vi "Stop Work.vi"(8 "error in (no error)":errorcluster, 9 "Reply":bool=TRUE, 10 "Reply to":refnum<class "Stop Response Msg.lvclass">, 11 "Measure Object in":refnum<class "Instrument Actor.lvclass">) -> (0 "error out":errorcluster, 3 "Measure Object out":refnum<class "Instrument Actor.lvclass">)   [LabVIEW 2018, in "Instrument Actor.lvclass"]
uses:
  Instrument Actor.lvclass
  Controllers/Process Controller Messages/Stop Response Msg/Stop Response Msg.lvclass
  Instrument Actor.lvclass/Instrument Actor.ctl
  Read Instrument driver.vi
  Write Instrument driver.vi
  NHMFL_Core/Libraries/Instruments/Instrument Driver/Instrument Driver.lvclass
  Worker/Worker.lvclass
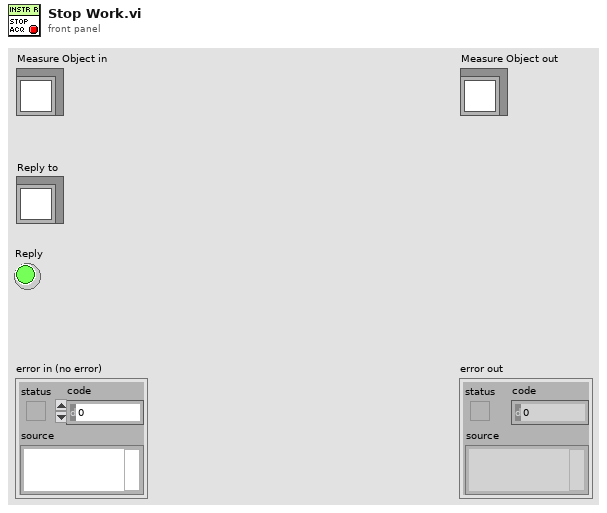
[diagram p1: front panel]
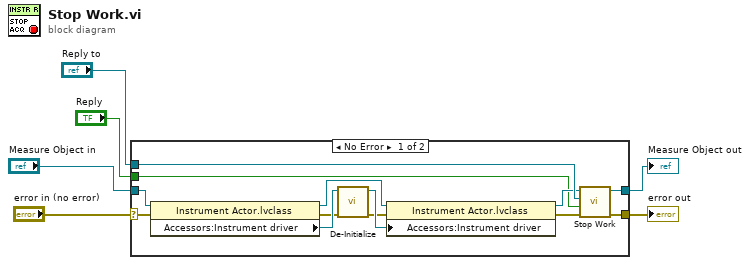
[diagram p0: block diagram]
diagram:
  n1 = case shown="No Error" "error in (no error)" {
    selector: "error in (no error)" -> [w7 w21]
    tunnel: [w19 w21] -> w6
    tunnel: [w18 w20] -> w5
    tunnel: "Reply to" -> [w17 _]
    tunnel: "Measure Object in" -> [w16 w20]
    tunnel: "Reply" -> [w8 _]
    frame No Error {
      n2 = property class="Instrument Actor.lvclass"(reference=w16, error in=w7) -> (reference out=w10:refnum<class "Instrument Actor.lvclass">, error out=w9:errorcluster, "Accessors:Instrument driver"=w15:refnum<class "Instrument Driver.lvclass">)
      n3 = call-dynamic "De-Initialize.vi"("error in (no error)"=w9, "Instrument Driver in"=w15) -> ("error out"=w13:errorcluster, "Instrument Driver out"=w14:refnum<class "Instrument Driver.lvclass">)  [unwired: 8 in]
      n4 = property class="Instrument Actor.lvclass"(reference=w10, error in=w13, "Accessors:Instrument driver"=w14) -> (reference out=w11:refnum<class "Instrument Actor.lvclass">, error out=w12:errorcluster)
      n5 = call-parent "Stop Work.vi"("error in (no error)"=w12, "Reply"=w8, "Reply to"=w17, "Measure Object in"=w11) -> ("error out"=w19:errorcluster, "Measure Object out"=w18:refnum<class "Instrument Actor.lvclass">)  [unwired: 6 in]
    }
    frame Error {
    }
  }
  "error out" <- w6
  "Measure Object out" <- w5
